vi "sync_alex_iteration.vi"(5 "frame number":i64, 6 "error in":errorcluster, 7 "data value reference":refnum<data-value>, 8 "last frame (s)":dbl, 9 "DAQmx Task":refnum<k21>) -> (0 "error out":errorcluster, 1 "Stop?":bool, 2 "relative seconds 2":dbl, 3 "task out":refnum<k21>)   [LabVIEW 2018, in "Synchronization Device.lvlib" / "Synchronization Device.lvclass"]
uses:
  Synchronization Device.lvclass
  <vilib>/DAQmx/write.llb/DAQmx Write (Digital 1D Bool 1Chan 1Samp).vi
  <vilib>/DAQmx/miscellaneous.llb/DAQmx Fill In Error Info.vi
panel:
  out "x .or. y?":bool
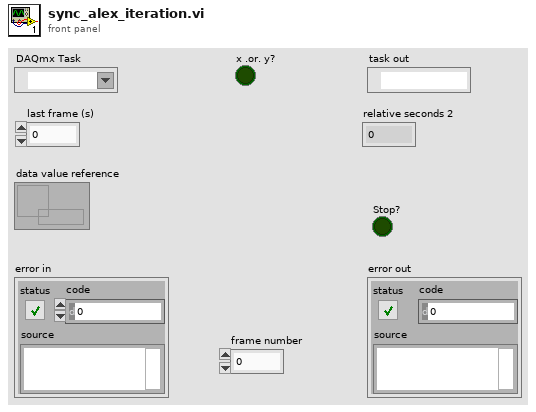
[diagram p1: front panel]
types:
  T1 = cluster{"Interval (ms)":dbl, "ALEX":bool, "Shutter Enable":bool[], "Stream":bool, "Duty Cycle":dbl}
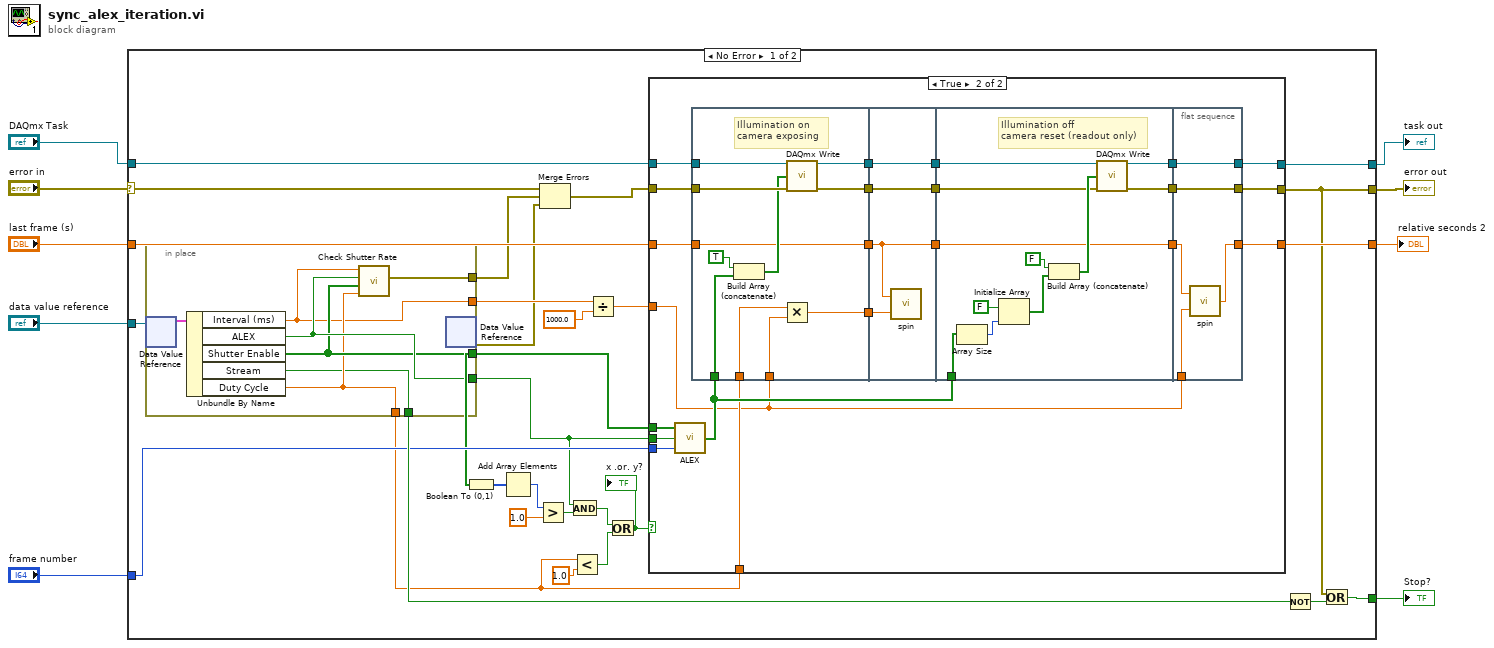
[diagram p0: block diagram]
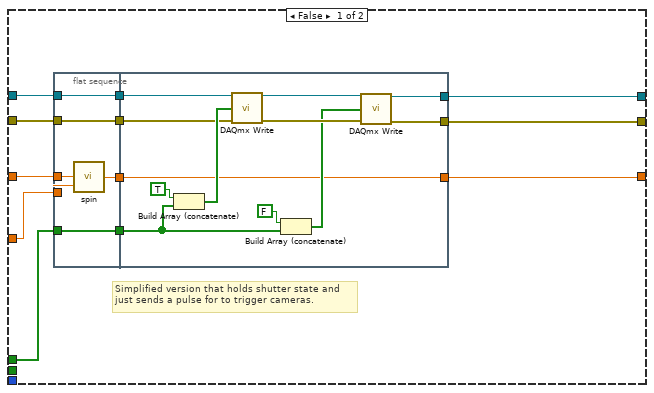
[diagram p2: hidden frame]
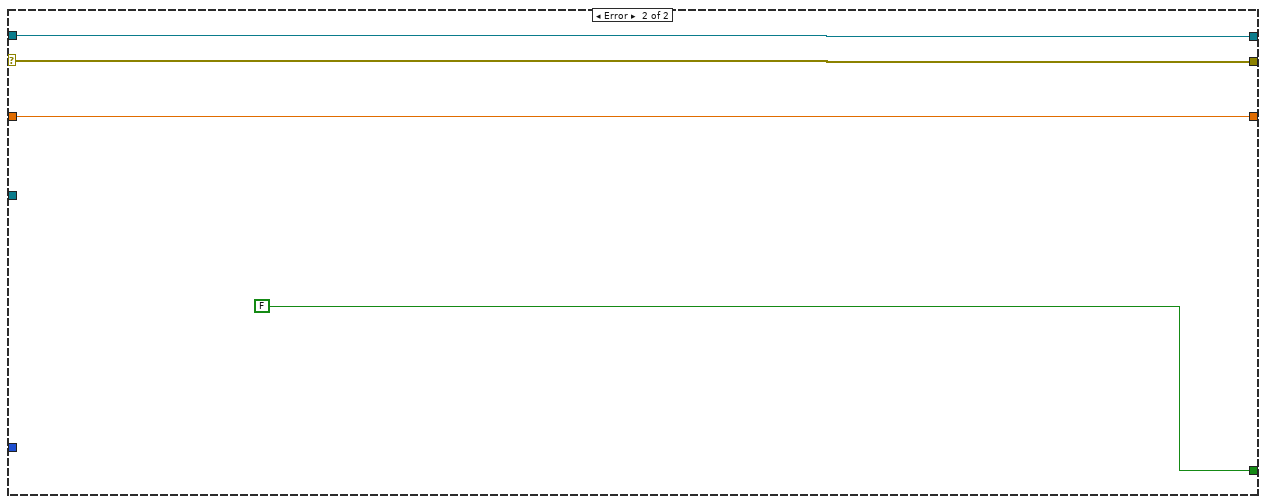
[diagram p3: hidden frame]
diagram:
  n1 = case shown="No Error" "error in" {
    selector: "error in" -> [w29 w129]
    tunnel: "DAQmx Task" -> [w37 w131]
    tunnel: [w36 w131] -> w8
    tunnel: [w26 w129] -> w7
    tunnel: "last frame (s)" -> [w35 w130]
    tunnel: [w34 w130] -> w5
    tunnel: "frame number" -> [w23 _]
    tunnel: "data value reference" -> [w30 _]
    tunnel: [w27 FALSE] -> w2
    frame No Error {
      n2 = in-place {
        in-place-border: [w38] -> w33
        in-place-border: [w42] -> w14
        in-place-border: [w40] -> w24
        in-place-border: [w43] -> w19
        in-place-border: [w41] -> w12
        in-place-border: [w39] -> w10
        n3 = in-place-dvr #1(w30) -> (w44:T1)  [unwired: 1 out]
        n4 = Unbundle By Name(w44) -> ("Interval (ms)"=w38:dbl, "ALEX"=w43:bool, "Shutter Enable"=w42:bool[], "Stream"=w40:bool, "Duty Cycle"=w41:dbl)
        n5 = call "Check Shutter Rate.vi"("Duty Cycle"=w41, "Shutter Enable"=w42, "ALEX"=w43, "Interval (ms)"=w38) -> ("error constant"=w39:errorcluster)  [unwired: 7 in]
        n6 = in-place-dvr #1() -> (w11:errorcluster)  [unwired: 1 in, 1 out]
      }
      n7 = Boolean To (0,1)(Boolean=w14) -> (0, 1=w15:i16[])
      n8 = Add Array Elements(numeric array=w15) -> (sum=w16:i16)
      n9 = Greater?(x=w16, y=1.0) -> (0:w18:bool)
      n10 = Merge Errors(w29, w10, w11) -> (w28:errorcluster)
      n11 = And(x=w19, y=w18) -> (x .and. y?=w20:bool)
      n12 = Less?(x=w12, y=1.0 ("x")) -> (x < y?=w21:bool)
      n13 = Divide(x=w33, y=1000.0) -> (x/y=w31:dbl)
      n14 = Or(x=w20, y=w21) -> (x .or. y?=w22:bool)
      "x .or. y?" <- w22
      n15 = case shown="True" w22 {
        tunnel: w37 -> [w54 w86]
        tunnel: [w56 w76] -> w36
        tunnel: w35 -> [w47 w78]
        tunnel: [w45 w85] -> w34
        tunnel: w12 -> [_ w79]
        tunnel: w31 -> [w48 w77]
        tunnel: w28 -> [w53 w84]
        tunnel: [w55 w75] -> w26
        tunnel: w23 -> [_ w83]
        tunnel: w19 -> [_ w82]
        tunnel: w14 -> [w52 w81]
        frame False {
          # "Simplified version that holds shutter state and\njust sends a pulse for to trigger cameras."
          n16 = flat-sequence {
            tunnel: w52 -> [w60]
            tunnel: w53 -> [w61]
            tunnel: w54 -> [w62]
            tunnel: [w62] -> w51
            tunnel: [w61] -> w50
            tunnel: [w60] -> w49
            tunnel: w48 -> [w59]
            tunnel: w47 -> [w58]
            tunnel: [w57] -> w46
            tunnel: [w72] -> w56
            tunnel: [w70] -> w55
            tunnel: w51 -> [w68]
            tunnel: w50 -> [w67]
            tunnel: w49 -> [w65]
            tunnel: w46 -> [w63]
            tunnel: [w63] -> w45
            frame #0 {
              n17 = call "spin.vi"("Interval"=w59, "relative seconds"=w58) -> ("relative seconds 2"=w57:dbl)
            }
            frame #1 {
              n18 = Build Array (concatenate)(TRUE, w65) -> (w73:bool[])
              n19 = call-poly <vilib>:"DAQmx Write.vi"("task/channels in"=w68, "data"=w73, "error in"=w67) -> ("task out"=w71:refnum<k21>, "error out"=w69:errorcluster)  [unwired: 10 in, 1 out]
              n20 = Build Array (concatenate)(FALSE, w65) -> (w64:bool[])
              n21 = call-poly <vilib>:"DAQmx Write.vi"("task/channels in"=w71, "data"=w64, "error in"=w69) -> ("task out"=w72:refnum<k21>, "error out"=w70:errorcluster)  [unwired: 10 in, 1 out]
            }
          }
        }
        frame True {
          n22 = call "ALEX.vi"("Frame Number"=w83, "ALEX?"=w82, "Shutter Enable"=w81) -> ("Shutter State"=w80:bool[])
          n23 = flat-sequence {
            tunnel: [w106] -> w96
            tunnel: [w98] -> w95
            tunnel: [w104] -> w94
            tunnel: w80 -> [w102]
            tunnel: w79 -> [w99]
            tunnel: w77 -> [w100]
            tunnel: [w97] -> w93
            tunnel: w86 -> [w107]
            tunnel: w84 -> [w105]
            tunnel: w78 -> [w98]
            tunnel: w96 -> [w111]
            tunnel: [w111] -> w92
            tunnel: w95 -> [w108]
            tunnel: [w108] -> w91
            tunnel: w94 -> [w110]
            tunnel: [w110] -> w90
            tunnel: w93 -> [w109]
            tunnel: w92 -> [w119]
            tunnel: w91 -> [w116]
            tunnel: w90 -> [w118]
            tunnel: [w117] -> w89
            tunnel: [w120] -> w88
            tunnel: w80 -> [w113]
            tunnel: [w116] -> w87
            tunnel: w89 -> [w123]
            tunnel: w88 -> [w124]
            tunnel: w77 -> [w127]
            tunnel: w87 -> [w126]
            tunnel: [w125] -> w85
            tunnel: [w124] -> w76
            tunnel: [w123] -> w75
            frame #0 {
              # "Illumination on\ncamera exposing"
              n24 = Build Array (concatenate)(TRUE, w102) -> (w101:bool[])
              n25 = Multiply(x=w99, y=w100) -> (x*y=w97:dbl)
              n26 = call-poly <vilib>:"DAQmx Write.vi"("task/channels in"=w107, "data"=w101, "error in"=w105) -> ("task out"=w106:refnum<k21>, "error out"=w104:errorcluster)  [unwired: 10 in, 1 out]
            }
            frame #1 {
              n27 = call "spin.vi"("Interval"=w109, "relative seconds"=w108) -> ()  [unwired: 1 out]
            }
            frame #2 {
              # "Illumination off\ncamera reset (readout only)"
              n28 = Array Size(array=w113) -> (size(s)=w115:i32)
              n29 = Initialize Array(FALSE, w115) -> (w112:bool[])
              n30 = Build Array (concatenate)(FALSE, w112) -> (w121:bool[])
              n31 = call-poly <vilib>:"DAQmx Write.vi"("task/channels in"=w119, "data"=w121, "error in"=w118) -> ("task out"=w120:refnum<k21>, "error out"=w117:errorcluster)  [unwired: 10 in, 1 out]
            }
            frame #3 {
              n32 = call "spin.vi"("Interval"=w127, "relative seconds"=w126) -> ("relative seconds 2"=w125:dbl)
            }
          }
        }
      }
      n33 = Not(x=w24) -> (.not. x?=w25:bool)
      n34 = Or(x=w26, y=w25) -> (x .or. y?=w27:bool)
    }
    frame Error {
    }
  }
  "task out" <- w8
  "error out" <- w7
  "relative seconds 2" <- w5
  "Stop?" <- w2
